vi "Problem 5 - Smallest multiple.vi"(8 "error in (no error)":errorcluster) -> (0 "error out":errorcluster, 2 "Execution time (ms)":u32, 3 "Answer (LCM of integers from 1 to 20)":i32)   [LabVIEW 2021, in "Project Euler.lvlib"]
uses:
  Project Euler.lvlib
  Utilities/Numeric Utilities/Numeric Utilities.lvlib
  Utilities/Named Timers/Named Timers.lvlib
panel:
  # "Development\ncontrols/indicators useful for development and testing, but which are not outputs of the VI"
  # "Input\nInputs to the VI"
  # "Output\nOutputs of the VI"
  # "Description\n\nBlank VI with error handling case. \n\nSummarize the use of this VI in this space."
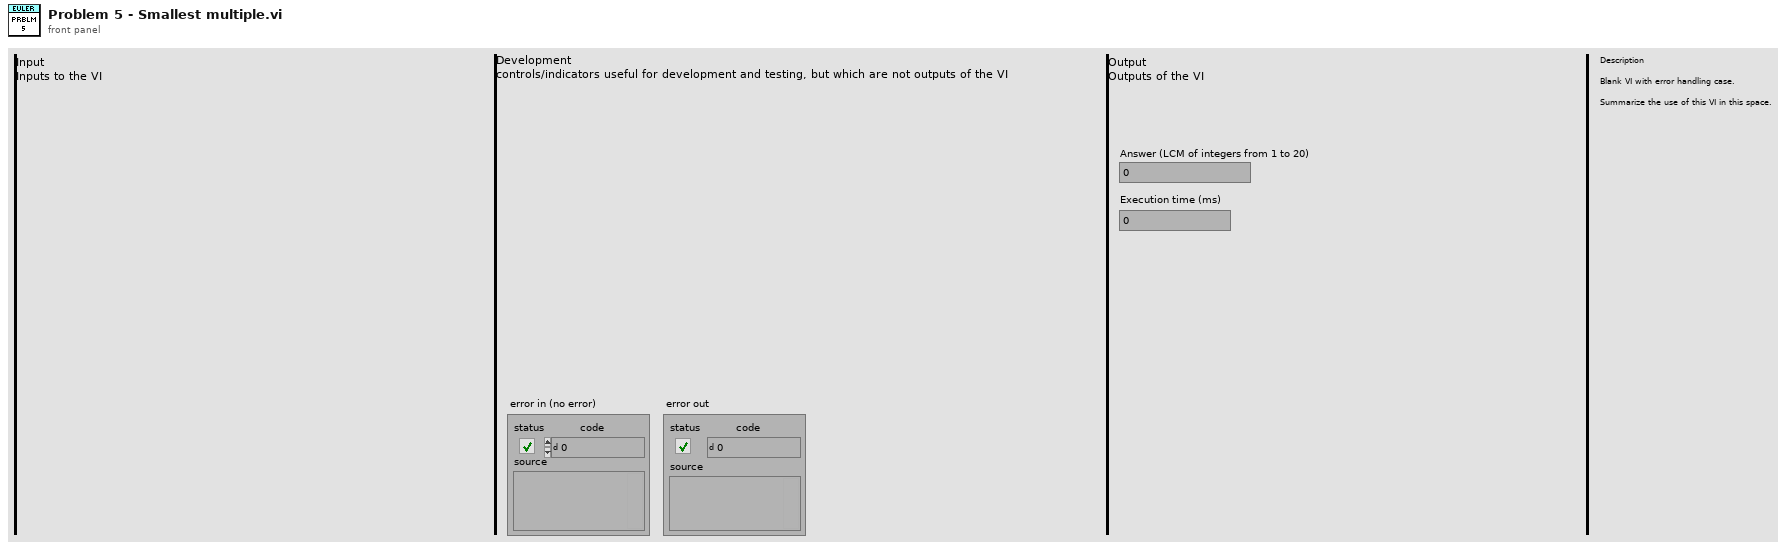
[diagram p1: front panel]
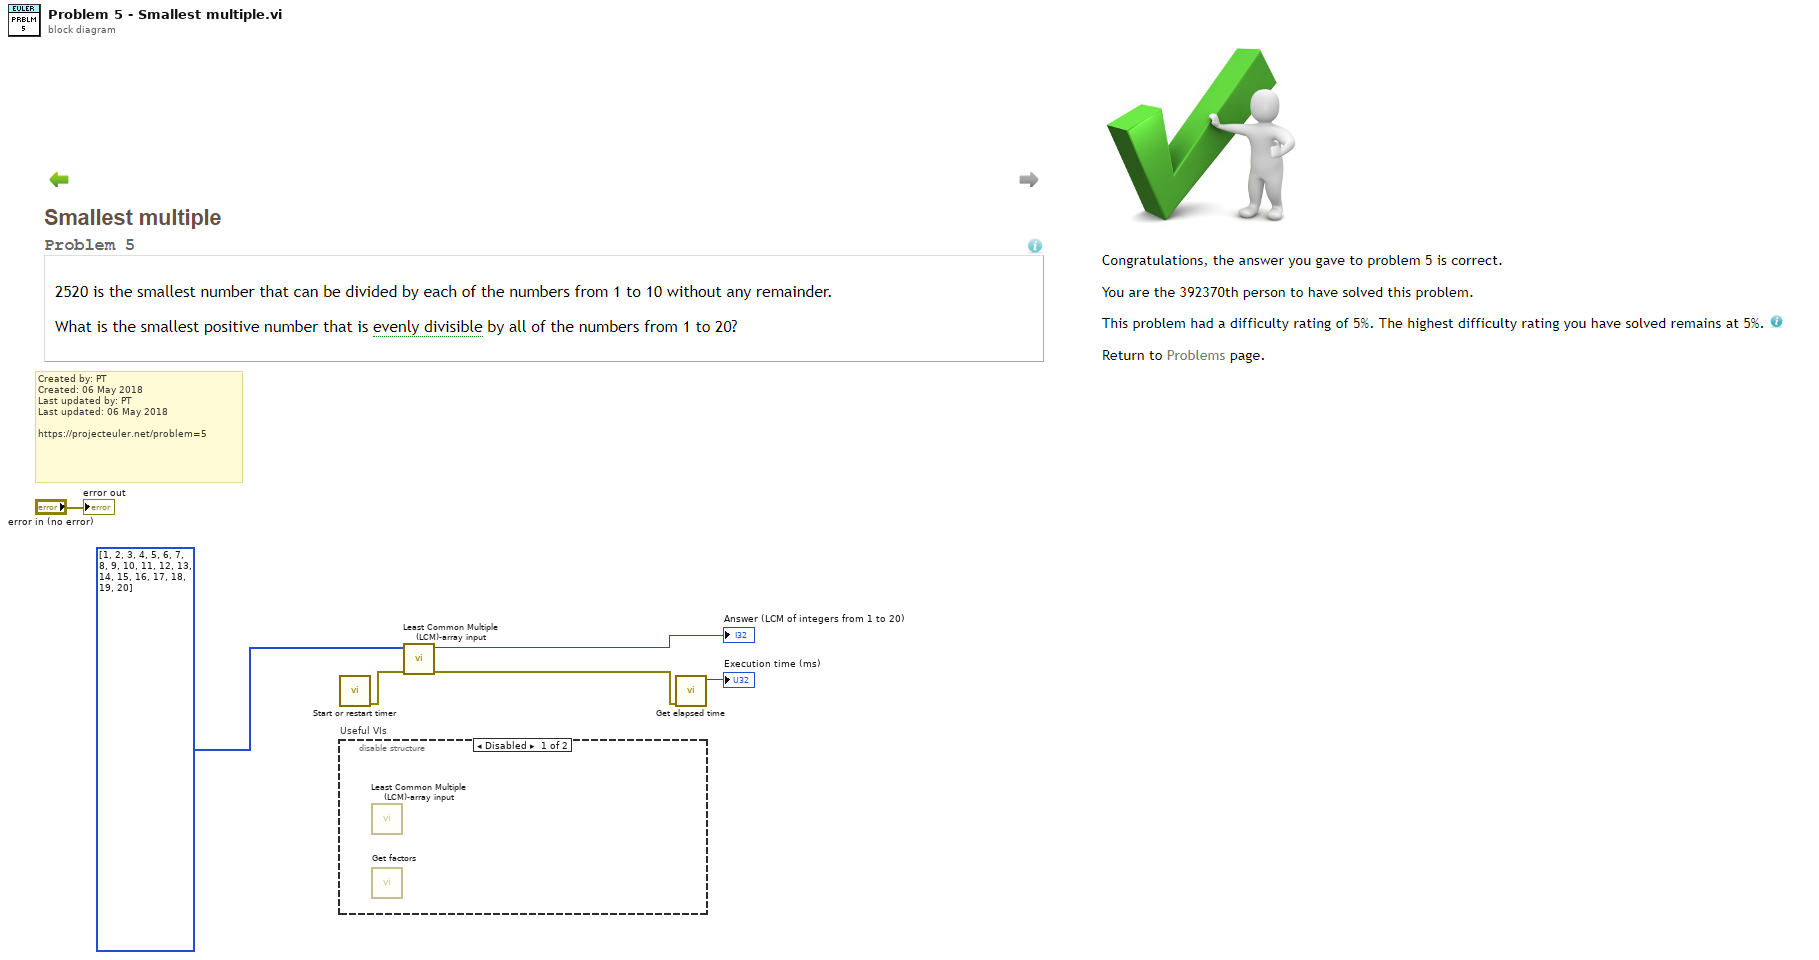
[diagram p0: block diagram]
diagram:
  # "Created by: PT\nCreated: 06 May 2018\nLast updated by: PT\nLast updated: 06 May 2018\n\nhttps://projecteuler.net/problem=5"
  n1 = call "Start or restart timer.vi"() -> ("error out"=w3:errorcluster)  [unwired: 11 in]
  n2 = disable-structure "Useful VIs" shown="Disabled" {
    frame Disabled {
      n3 = call "Least Common Multiple (LCM)-array input.vi"() -> ()  [unwired: 10 in, 2 out]
      n4 = call "Get factors.vi"() -> ()  [unwired: 6 in, 6 out]
    }
    frame Enabled {
    }
  }
  n5 = call "Least Common Multiple (LCM)-array input.vi"("error in (no error)"=w3, "Input integers"=i32[] [1, 2, 3, 4, 5, 6, 7, 8, 9, 10, 11, 12, 13, 14, 15, 16, 17, 18, 19, 20]) -> ("error out"=w2:errorcluster, "Least Common Multiple (LCM)"=→"Answer (LCM of integers from 1 to 20)":i32)  [unwired: 8 in]
  n6 = call "Get elapsed time.vi"("error in (no error)"=w2) -> ("Elapsed time (ms)"=→"Execution time (ms)":u32)  [unwired: 7 in, 3 out]
  "error out" <- "error in (no error)"
